vi "Lang Set Frame b.vi"(8 "error in (no error)":errorcluster, 10 "b":T1, 11 "LF2R IDE in":refnum<class "Main Panel.lvclass">) -> (0 "error out":errorcluster, 3 "LF2R IDE out":refnum<class "Main Panel.lvclass">)   [LabVIEW 2018, in "Main Panel.lvlib" / "Main Panel.lvclass"]
uses:
  Main Panel.lvclass
  Framework/Framework/Const Lang MainWnd Frame b.ctl
  Framework/Framework/Const Lang Property.ctl
  Main Panel.lvclass/Main Panel.ctl
  Framework/Framework/Framework.lvclass
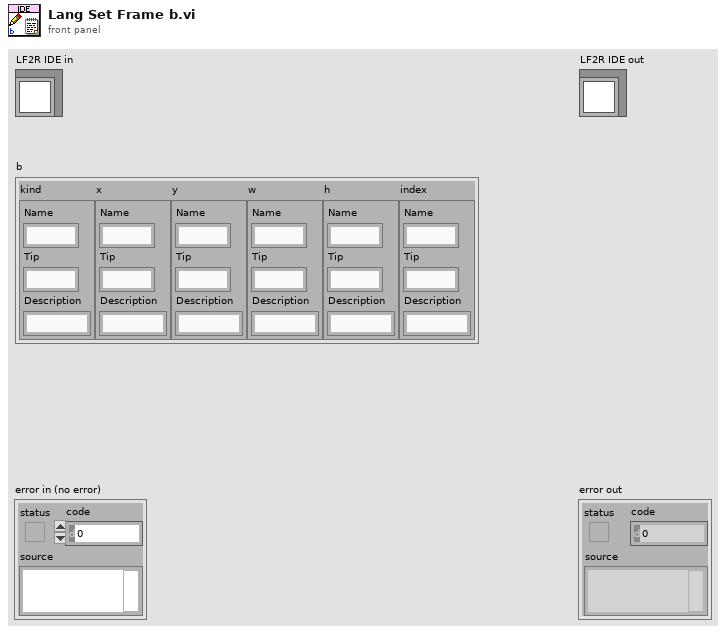
[diagram p1: front panel]
types:
  T1 = typedef "Framework.lvlib/Framework.lvclass/Const Lang MainWnd Frame b.ctl" = cluster{"kind":T2, "x":T2, "y":T2, "w":T2, "h":T2, "index":T2}
  T2 = typedef "Framework.lvlib/Framework.lvclass/Const Lang Property.ctl" = cluster{"Name":string, "Tip":string, "Description":string}
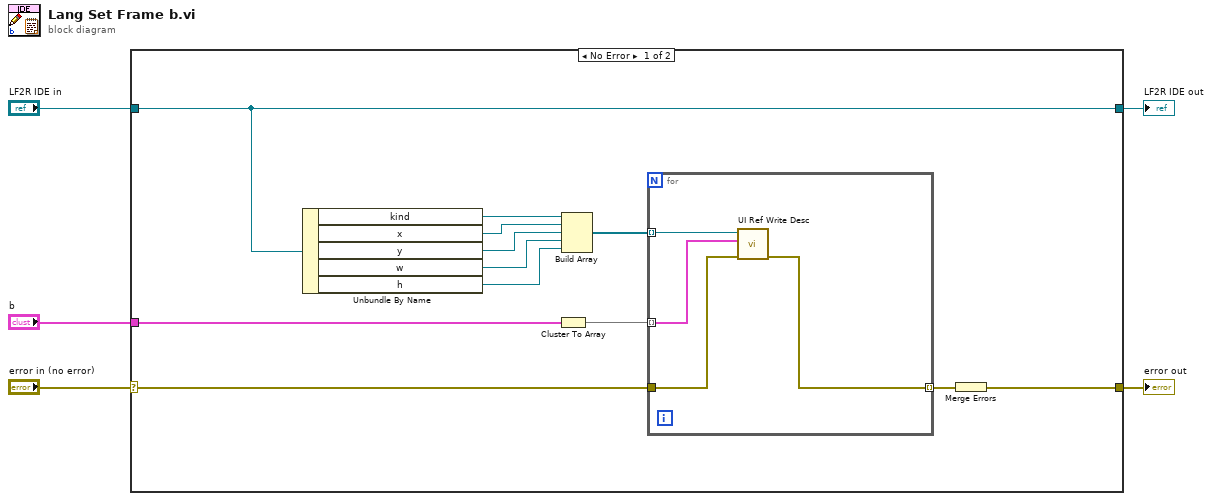
[diagram p0: block diagram]
diagram:
  n1 = case shown="No Error" "error in (no error)" {
    selector: "error in (no error)" -> [w13 w23]
    tunnel: [w11 w23] -> w4
    tunnel: [w17 w22] -> w2
    tunnel: "LF2R IDE in" -> [w17 w22]
    tunnel: "b" -> [w15 _]
    frame No Error {
      n2 = Unbundle By Name(w17) -> ("kind"=w10:refnum<vi>, "x"=w9:refnum<vi>, "y"=w8:refnum<vi>, "w"=w7:refnum<vi>, "h"=w6:refnum<vi>)
      n3 = Cluster To Array(cluster=w15) -> (array=w14:T2[])
      n4 = Build Array(w10, w9, w8, w7, w6) -> (w16:refnum<vi>[])
      n5 = for {
        tunnel: w16 -> [w18] mode=indexing
        tunnel: w14 -> [w21] mode=indexing
        tunnel: w13 -> [w20]
        tunnel: [w19] -> w12 mode=indexing
        n6 = call "UI Ref Write Desc.vi"("error in (no error)"=w20, "UI Property"=w21, "UI Ref"=w18) -> ("error out"=w19:errorcluster)  [unwired: 8 in]
      }
      n7 = Merge Errors(w12) -> (w11:errorcluster)
    }
    frame Error {
    }
  }
  "error out" <- w4
  "LF2R IDE out" <- w2
